vi "Init.vi"(8 "error in (no error)":errorcluster, 10 "Product_Ref":string, 11 "Board in":refnum<class "Motherboard.lvclass">) -> (0 "error out":errorcluster, 3 "Board out":refnum<class "Motherboard.lvclass">)   [LabVIEW 2025, in "SW License Manager.lvlib" / "Motherboard.lvclass"]
uses:
  Motherboard.lvclass
  <vilib>/Utility/error.llb/Error Cluster From Error Code.vi
  <vilib>/ErrorRing/Error Ring.xnode
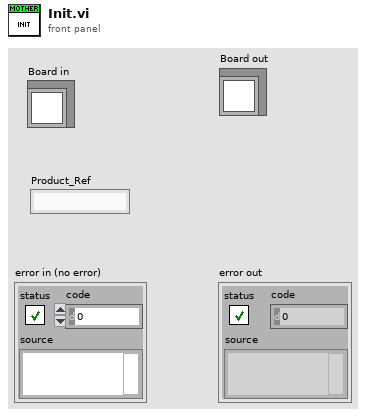
[diagram p1: front panel]
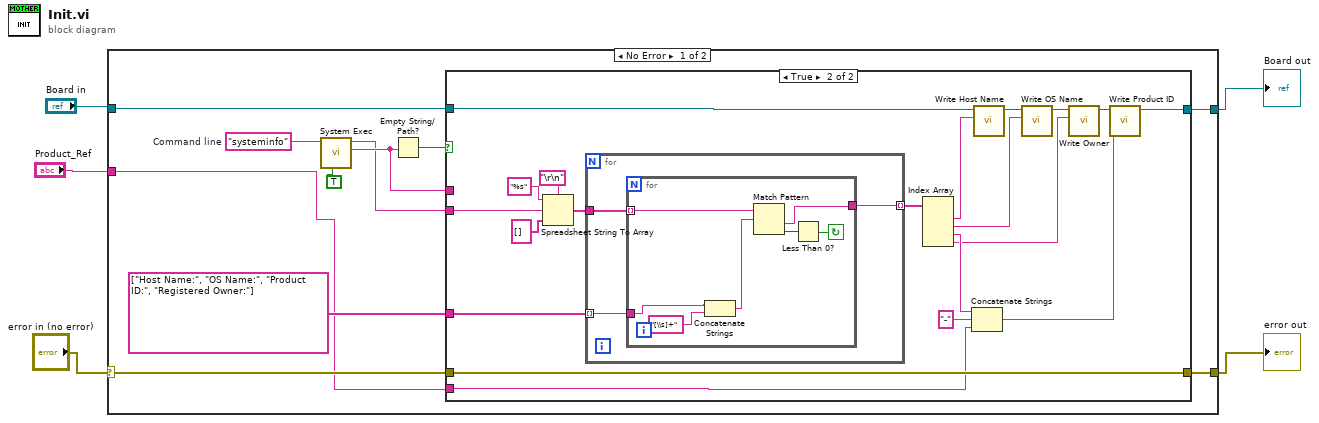
[diagram p0: block diagram]
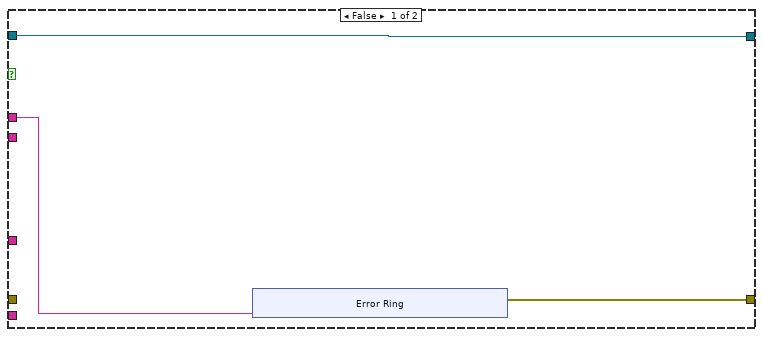
[diagram p2: hidden frame]
diagram:
  n1 = case shown="No Error" "error in (no error)" {
    selector: "error in (no error)" -> [w15 w58]
    tunnel: [w16 w58] -> w2
    tunnel: [w10 w57] -> w3
    tunnel: "Board in" -> [w9 w57]
    tunnel: "Product_Ref" -> [w6 _]
    frame No Error {
      w13 = "systeminfo"  # Command line
      n2 = call <vilib>:"System Exec.vi"("run minimized? (F)"=TRUE, "command line"=w13) -> ("standard error"=w12:string, "standard output"=w11:string)  [unwired: 6 in, 2 out]
      n3 = Empty String/Path?(string/path=w12) -> (empty?=w14:bool)
      n4 = case shown="True" w14 {
        tunnel: [w19 w46] -> w16
        tunnel: w15 -> [_ w46]
        tunnel: w12 -> [w18 _]
        tunnel: w11 -> [_ w41]
        tunnel: [w17 w31] -> w10
        tunnel: w9 -> [w17 w35]
        tunnel: string[] ["Host Name:", "OS Name:", "Product ID:", "Registered Owner:"] -> [_ w45]
        tunnel: w6 -> [_ w36]
        frame False {
          n5 = xnode "Error Ring"("parameter 0"=w18) -> ("error out"=w19:errorcluster)
        }
        frame True {
          n6 = Spreadsheet String To Array(delimiter (Tab)="\r\n", format string="%s" ("String"), spreadsheet string=w41, array type (2D Dbl)=string[] []) -> (array=w43:string[])
          n7 = for {
            tunnel: w45 -> [w49] mode=indexing
            tunnel: w43 -> [w48]
            tunnel: [w47] -> w39 mode=indexing
            n8 = for {
              tunnel: w49 -> [w56]
              tunnel: w48 -> [w53] mode=indexing
              tunnel: [w50] -> w47
              stop <- w51 continue-if-true
              n9 = Concatenate Strings(w56, "[\\s]+" ("string")) -> (w54:string)
              n10 = Match Pattern(string=w53, regular expression=w54) -> (after substring=w50:string, offset past match=w52:i32)  [unwired: 1 in, 2 out]
              n11 = Less Than 0?(x=w52) -> (x < 0?=w51:bool)
            }
          }
          n12 = Index Array(array=w39) -> (element #1=w27:string, element #2=w28:string, element #3=w38:string, element #4=w29:string)  [unwired: 4 in]
          n13 = Concatenate Strings(w38, "-" ("string"), w36) -> (w30:string)
          n14 = call-dynamic "Write Host Name.vi"("Host Name"=w27, "Board in"=w35) -> ("Board out"=w34:refnum<class "Motherboard.lvclass">)  [unwired: 8 in, 1 out]
          n15 = call-dynamic "Write OS Name.vi"("OS Name"=w28, "Board in"=w34) -> ("Board out"=w33:refnum<class "Motherboard.lvclass">)  [unwired: 8 in, 1 out]
          n16 = call-dynamic "Write Owner.vi"("Owner"=w29, "Board in"=w33) -> ("Board out"=w32:refnum<class "Motherboard.lvclass">)  [unwired: 8 in, 1 out]
          n17 = call-dynamic "Write Product ID.vi"("Product ID"=w30, "Board in"=w32) -> ("Board out"=w31:refnum<class "Motherboard.lvclass">)  [unwired: 8 in, 1 out]
        }
      }
    }
    frame Error {
    }
  }
  "error out" <- w2
  "Board out" <- w3
